vi "get.Length.vi"(8 "error in (no error)":errorcluster, 11 "PitchMessage in":refnum<class "PitchMessage.lvclass">) -> (0 "error out":errorcluster, 2 "Length":u16, 3 "PitchMessage out":refnum<class "PitchMessage.lvclass">)   [LabVIEW 2020, in "PitchMessage.lvclass"]
uses:
  PitchMessage.lvclass
  PitchMessage.lvclass/PitchMessage.ctl
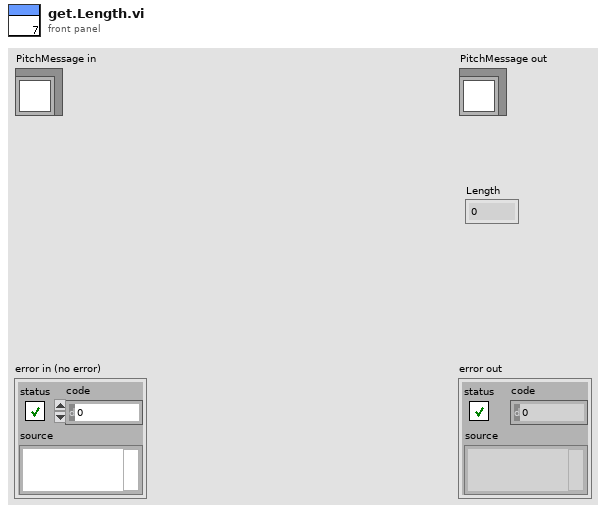
[diagram p1: front panel]
types:
  T1 = typedef "FieldValue.ctl" = variant
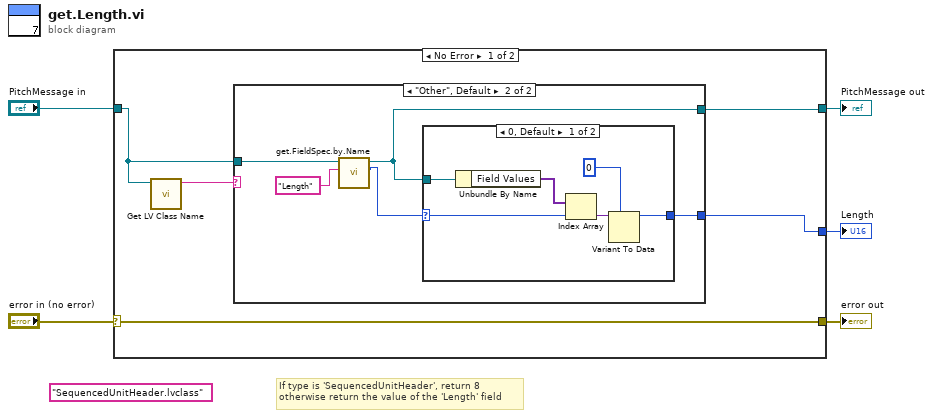
[diagram p0: block diagram]
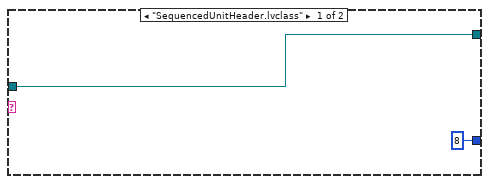
[diagram p2: hidden frame]
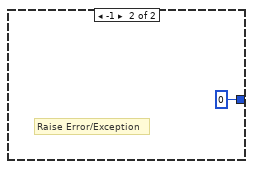
[diagram p3: hidden frame]
diagram:
  (unwired) "SequencedUnitHeader.lvclass"
  # "If type is 'SequencedUnitHeader', return 8\notherwise return the value of the 'Length' field"
  n1 = case shown="No Error" "error in (no error)" {
    selector: "error in (no error)" -> [w10 w26]
    tunnel: [w10 w26] -> w4
    tunnel: [w6 w25] -> w2
    tunnel: "PitchMessage in" -> [w8 w25]
    tunnel: [w9 _] -> w1
    frame No Error {
      n2 = call <vilib>:"Get LV Class Name.vi"("object"=w8) -> ("class name"=w7:string)  [unwired: 9 in, 1 out]
      n3 = case shown="\"Other\", Default" w7 {
        tunnel: [u16 8 w15] -> w9
        tunnel: w8 -> [w11 w14]
        tunnel: [w11 w13] -> w6
        frame "SequencedUnitHeader.lvclass" {
        }
        frame "Other", Default {
          n4 = call-dynamic "get.FieldSpec.by.Name.vi"("Field.Name"="Length", "PitchMessage in"=w14) -> ("Index"=w16:i32, "PitchMessage out"=w13:refnum<class "PitchMessage.lvclass">)  [unwired: 7 in, 1 out]
          n5 = case shown="0, Default" w16 {
            selector: w16 -> [w22 _]
            tunnel: w13 -> [w23 _]
            tunnel: [w18 u16 0] -> w15
            frame 0, Default {
              n6 = Unbundle By Name(w23) -> ("Field Values"=w21:T1[])
              n7 = Index Array(array=w21, index=w22) -> (element=w19:T1)
              n8 = Variant To Data(type=u16 0, Variant=w19) -> (data=w18:u16)  [unwired: 1 in, 1 out]
            }
            frame -1 {
              # "Raise Error/Exception"
            }
          }
        }
      }
    }
    frame Error {
    }
  }
  "error out" <- w4
  "PitchMessage out" <- w2
  "Length" <- w1
